vi "JKISM++ Registrer Status Change.vi"(0 "Source JKISM Name":string, 5 "Dest JKISM Name":string, 7 "Message":string, 9 "ActingMsg (\"\" to use Message)":string, 11 "Error in":errorcluster caption="Error in (no error)") -> (4 "Source JKISM Name(dup)":string, 15 "Error out":errorcluster)   [LabVIEW 2014, in "JKI-State-Machine-Plus.lvlib"]
uses:
  JKI-State-Machine-Plus.lvlib
  _Support/FGV-BroadcastRegistry/Oper-BroadcastRegistry.ctl
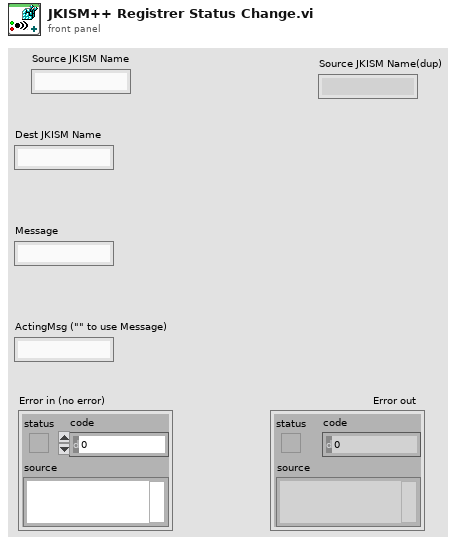
[diagram p1: front panel]
types:
  T1 = typedef "JKI-State-Machine-Plus.lvlib/Oper-BroadcastRegistry.ctl" = enum16{"Delete Source Module", "Delete Dest Module", "Remove Module", "Register", "Unregister", "Check"}
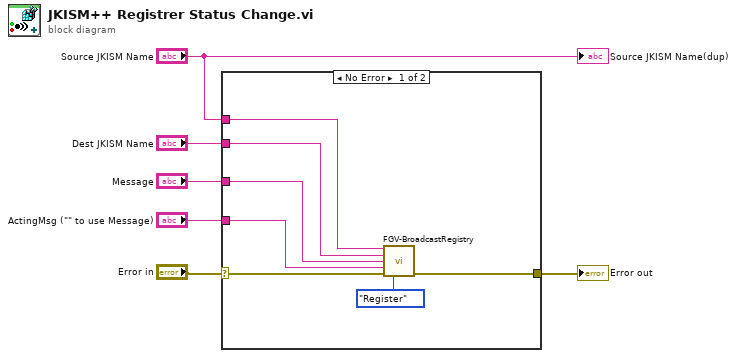
[diagram p0: block diagram]
diagram:
  n1 = case shown="No Error" "Error in" {
    selector: "Error in" -> [w12 w14]
    tunnel: [w11 w14] -> w5
    tunnel: "ActingMsg (\"\" to use Message)" -> [w10 _]
    tunnel: "Message" -> [w9 _]
    tunnel: "Dest JKISM Name" -> [w8 _]
    tunnel: "Source JKISM Name" -> [w7 _]
    frame No Error {
      n2 = call "FGV-BroadcastRegistry.vi"("Source"=w7, "Dest"=w8, "Message"=w9, "ActingMsg In"=w10, "Error in"=w12, "Operation"=Oper-BroadcastRegistry."Register") -> ("Error out"=w11:errorcluster)  [unwired: 8 in, 1 out]
    }
    frame Error {
    }
  }
  "Error out" <- w5
  "Source JKISM Name(dup)" <- "Source JKISM Name"
